vi "UI Traverse Curr File.vi"(7 "Tot Files":refnum<vi>, 8 "error in (no error)":errorcluster, 9 "Current File in":i32, 10 "File Paths":path[](array[path]), 11 "Slide in":refnum<vi>) -> (0 "error out":errorcluster)   [LabVIEW 2020, in "DocTool.lvlib"]
uses:
  DocTool.lvlib
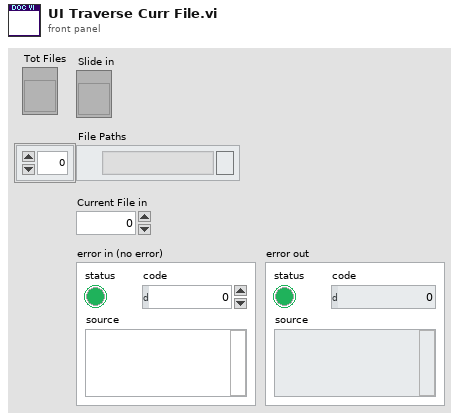
[diagram p1: front panel]
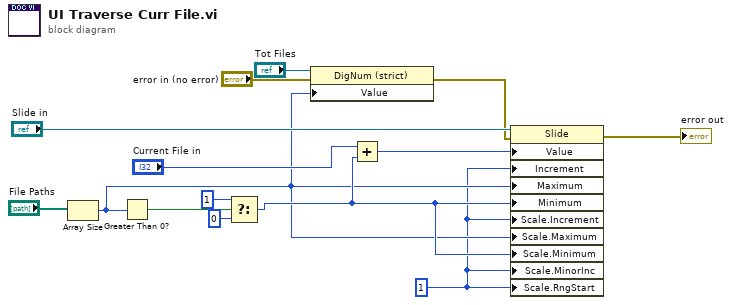
[diagram p0: block diagram]
diagram:
  w1 = 1 ("t")
  n1 = Array Size(array="File Paths") -> (size(s)=w2:i32)
  n2 = Greater Than 0?(x=w2) -> (x > 0?=w13:bool)
  n3 = Select(t=1, s=w13, f=0 ("t")) -> (s? t:f=w6:i32)
  n4 = property class="DigNum (strict)"(reference="Tot Files", error in="error in (no error)", "Value"=w2) -> (error out=w3:errorcluster)  [unwired: 1 out]
  n5 = Add(x="Current File in", y=w6) -> (x+y=w11:i32)
  n6 = property class="Slide"(reference="Slide in", error in=w3, "Value"=w11, "Increment"=w1, "Maximum"=w2, "Minimum"=w6, "Scale.Increment"=w1, "Scale.Maximum"=w2, "Scale.Minimum"=w6, "Scale.MinorInc"=w1, "Scale.RngStart"=w1) -> (error out=→"error out":errorcluster)  [unwired: 1 out]
